vi "booleans to data.vi"(9 "specifications":T1[](array[typedef]), 10 "booleans":bool[](array[boolean]), 11 "allocation":T3) -> (3 "data table":T3)   [LabVIEW 2015, in "Modbus Module runtime.lvclass"]
uses:
  Modbus Module runtime.lvclass
  <vilib>/NI/Tag Bus/table/data table.ctl
  data mapping elements.ctl
  <vilib>/NI/Tag Bus/tag/Data Type.ctl
  <vilib>/NI/Tag Bus/table/data polymorphs/write one/write Boolean.vi
  <vilib>/NI/Tag Bus/table/data table.lvlib
  <vilib>/NI/Tag Bus/tag/tag descriptor.lvclass
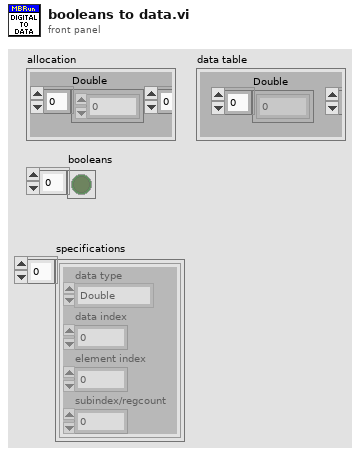
[diagram p1: front panel]
types:
  T1 = typedef "Modbus Module runtime.lvclass/data mapping elements.ctl" = cluster{"data type":T2, "data index":i32, "element index":i32, "subindex/regcount":i32}
  T2 = typedef "tag bus.lvlib/tag descriptor.lvclass/Data Type.ctl" = enum16{"Double", "Single", "I64", "I32", "I16", "I8", "U64", "U32", "U16", "U8", "Boolean", "String", "Array of Double", "Array of Single", "Array of I64", "Array of I32", "Array of I16", "Array of I8", "Array of U64", "Array of U32", "Array of U16", "Array of U8", "Array of Boolean", "Array of String"}
  T3 = typedef "tag bus.lvlib/data table.lvlib/data table.ctl" = cluster{"Double":dbl[], "Single":sgl[], "I64":i64[], "I32":i32[], "I16":i16[], "I8":i8[], "U64":u64[], "U32":u32[], "U16":u16[], "U8":u8[], "Boolean":bool[], "String":string[], "Array of Double":cluster{"DBL Array":dbl[]}[], "Array of Single":cluster{"SGL Array":sgl[]}[], "Array of I64":cluster{"I64 Array":i64[]}[], "Array of I32":cluster{"I32 Array":i32[]}[], "Array of I16":cluster{"I16 Array":i16[]}[], "Array of I8":cluster{"I8 Array":i8[]}[], "Array of U64":cluster{"U64 Array":u64[]}[], "Array of U32":cluster{"U32 Array":u32[]}[], "Array of U16":cluster{"U16 Array":u16[]}[], "Array of U8":cluster{"U8 Array":u8[]}[], "Array of Boolean":cluster{"Boolean Array":bool[]}[], "Array of String":cluster{"String Array":string[]}[]}
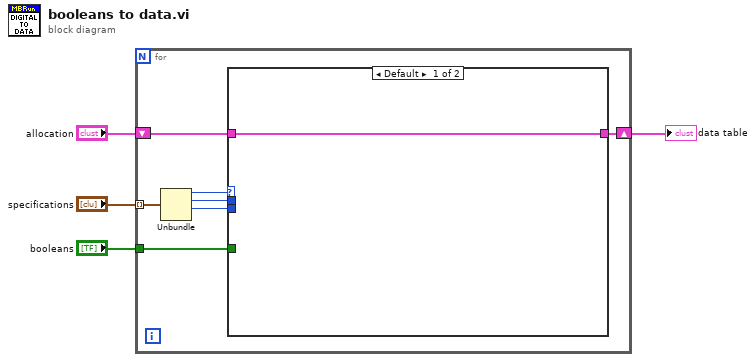
[diagram p0: block diagram]
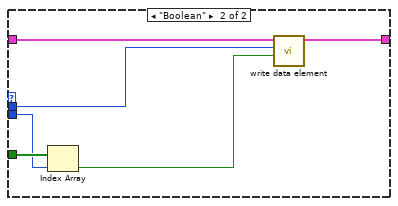
[diagram p2: hidden frame]
diagram:
  n1 = for {
    shift-right: [w8] -> w3
    shift-left: "allocation" -> [w9]
    tunnel: "booleans" -> [w7]
    tunnel: "specifications" -> [w11] mode=indexing
    n2 = Unbundle(w11) -> ("data type"=w10:T2, "data index"=w6:i32, "element index"=w5:i32)  [unwired: 1 out]
    n3 = case shown="Default" w10 {
      tunnel: w9 -> [w12 w18]
      tunnel: [w12 w17] -> w8
      tunnel: w5 -> [_ w15]
      tunnel: w7 -> [_ w16]
      tunnel: w6 -> [_ w14]
      frame Default {
      }
      frame "Boolean" {
        n4 = Index Array(array=w16, index=w15) -> (element=w13:bool)
        n5 = call-poly <vilib>:"write data element.vi"("value"=w13, "index"=w14, "data table in"=w18) -> ("data table out"=w17:T3)  [unwired: 8 in]
      }
    }
  }
  "data table" <- w3
